vi "Get Robot Competition Mode.vi"(8 "Right Auton Limit":dbl, 9 "Right Teleop Limit":dbl, 10 "Finish":bool, 11 "DS Occurrence":refnum<k4>) -> (0 "Match Info out":T1={"Autonomous Elapsed Seconds"=0.0, "TeleOp Elapsed Seconds"=0.0, "Disabled Elapsed Seconds"=0.0, "Visited Autonomous"=FALSE, "Visited TeleOp"=FALSE, "Visited Disabled"=FALSE, "Autonomous Settings"={"Autonomous Style"=enum."Independent", "VI Refnum"=refnum}}, 1 "RawControlByte":u8 format="%08b", 2 "Call Context":T2, 3 "Robot Mode":T3, 4 "Right Limit":dbl)   [LabVIEW 2011]
doc: "<b>Get Competition Mode.vi</b> returns the mode of the current phase of competition, which determines the current restrictions of robot operation that apply. Possible modes include <b>Autonomous Disabled</b>, <b>Autonomous Enabled</b>, <b>Teleop Disabled</b>, and <b>Teleop Enabled</b>.\n\nThis software is licensed. Open the labview\\readme\\WPI Robotics Library Open Source License.txt file for more information."
uses:
  <vilib>/Rock Robotics/WPI/DriverStation/WPI_DriverStationRobotMode.ctl
  <vilib>/Rock Robotics/WPI/DriverStation/WPI_DriverStationDerivedRobotMode.ctl
  <vilib>/Rock Robotics/WPI/DriverStation/WPI_DriverStationMatch Info.ctl
  <vilib>/Rock Robotics/WPI/DriverStation/WPI_DriverStationCommDataCacheOp.ctl
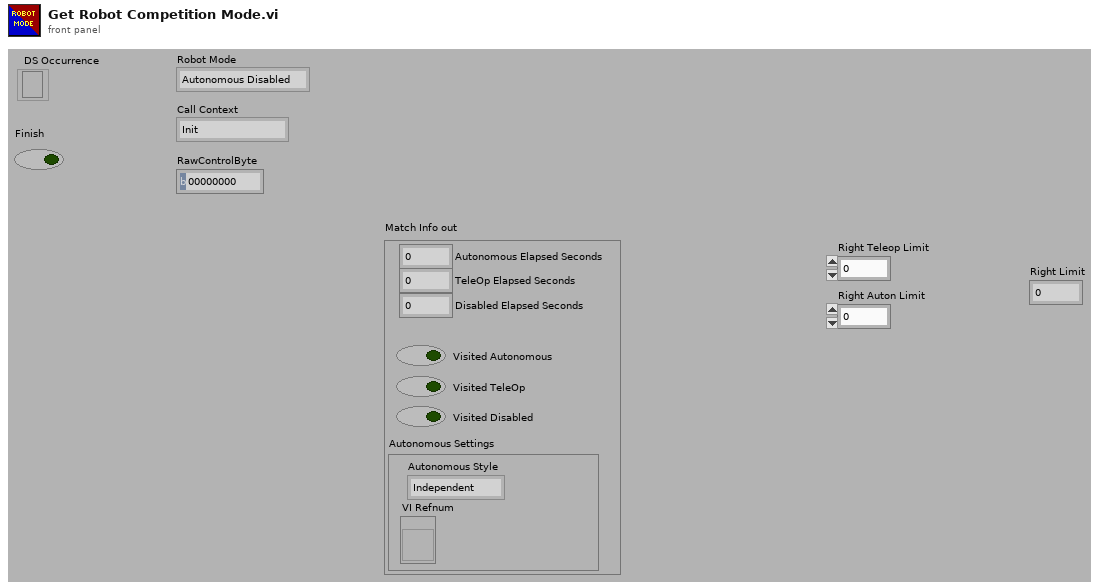
[diagram p1: front panel]
types:
  T1 = typedef "WPI_DriverStationMatch Info.ctl" = cluster{"Autonomous Elapsed Seconds":dbl, "TeleOp Elapsed Seconds":dbl, "Disabled Elapsed Seconds":dbl, "Visited Autonomous":bool, "Visited TeleOp":bool, "Visited Disabled":bool, "Autonomous Settings":cluster{"Autonomous Style":enum16{"Iterative", "Independent"}, "VI Refnum":refnum<vi>}}
  T2 = typedef "WPI_DriverStationDerivedRobotMode.ctl" = enum16{"Init", "Execute", "Stop"}
  T3 = typedef "WPI_DriverStationRobotMode.ctl" = enum16{"Autonomous Disabled", "Autonomous Enabled", "Teleop Disabled", "Teleop Enabled", "Timeout", "Finish"}
  T4 = typedef "WPI_DriverStationCommDataCacheOp.ctl" = enum16{"Get", "Set", "Init"}
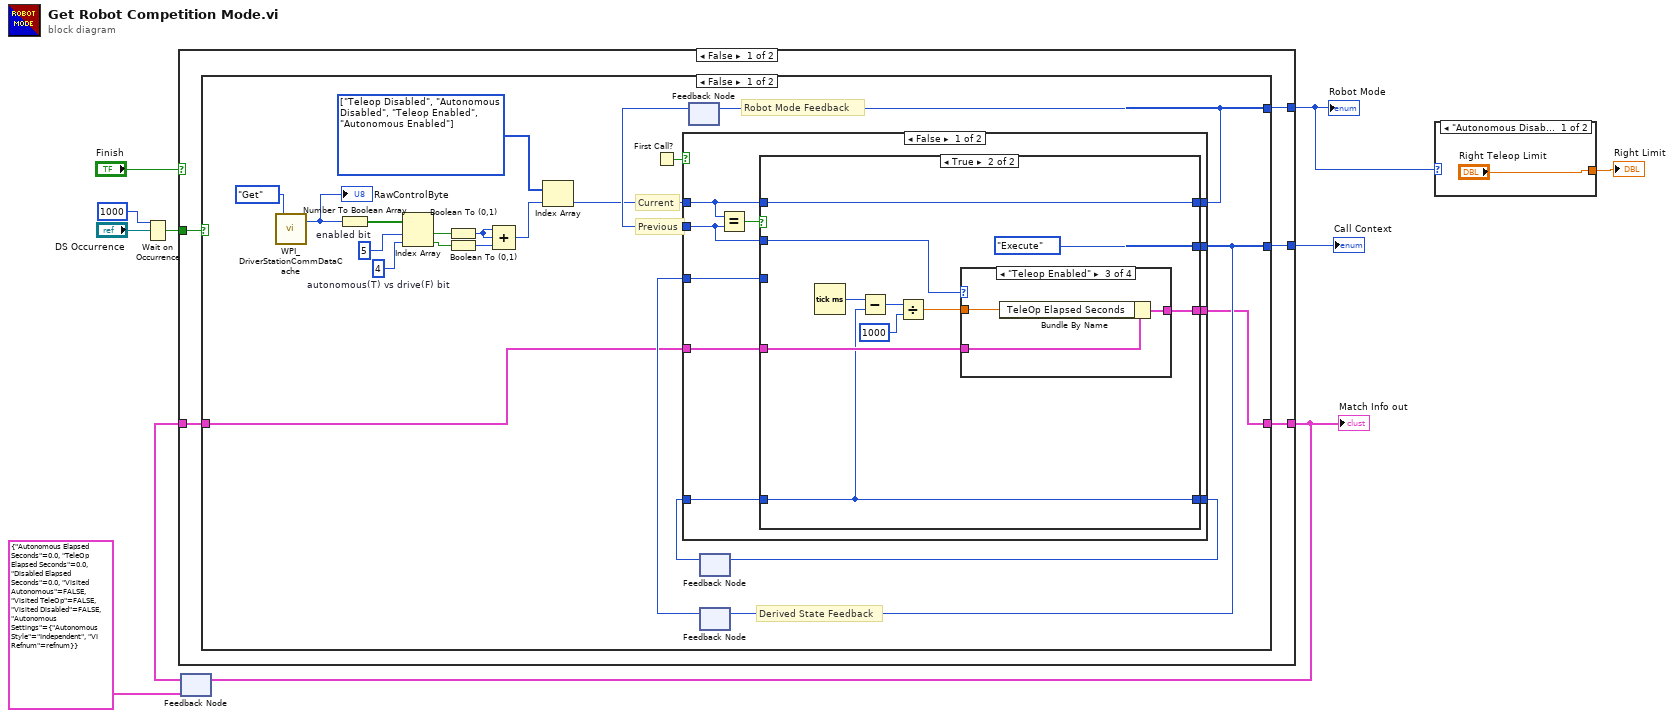
[diagram p0: block diagram]
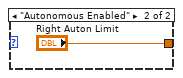
[diagram p2: hidden frame]
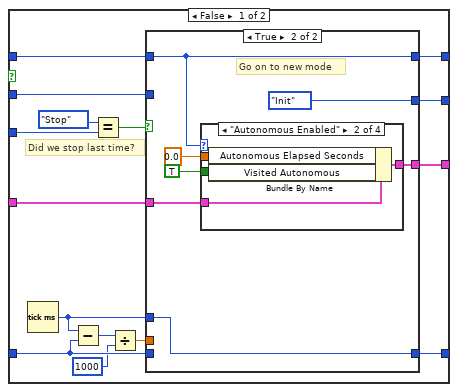
[diagram p3: hidden frame]
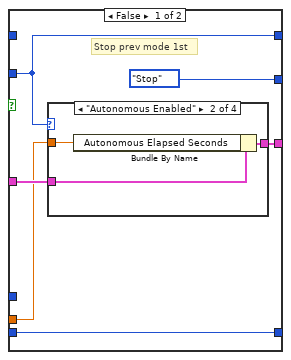
[diagram p4: hidden frame]
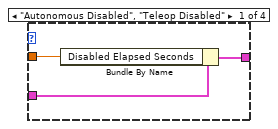
[diagram p5: hidden frame]
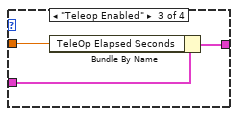
[diagram p6: hidden frame]
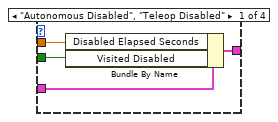
[diagram p8: hidden frame]
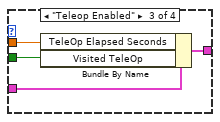
[diagram p9: hidden frame]
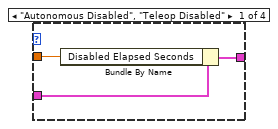
[diagram p11: hidden frame]
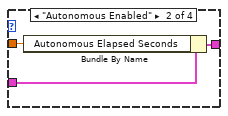
[diagram p12: hidden frame]
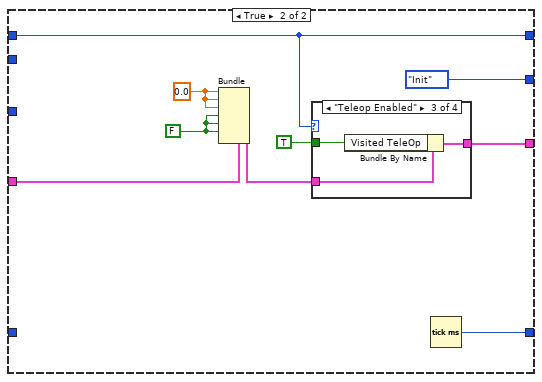
[diagram p14: hidden frame]
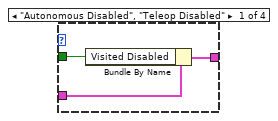
[diagram p15: hidden frame]
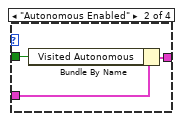
[diagram p16: hidden frame]
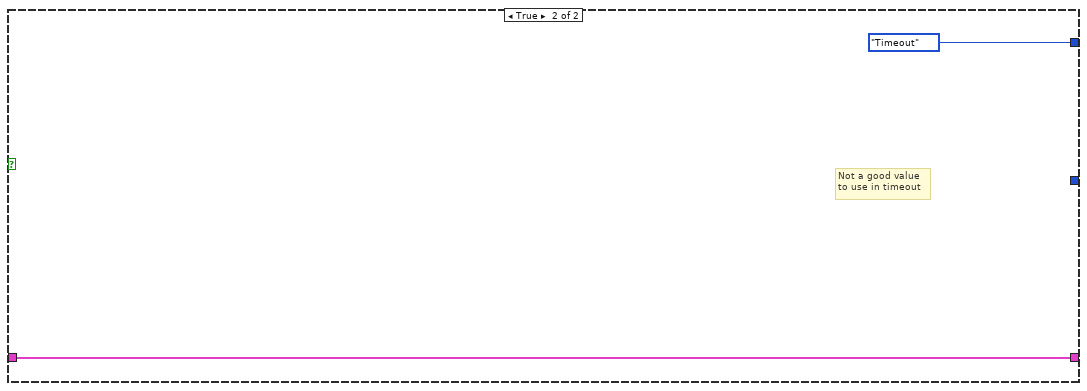
[diagram p18: hidden frame]
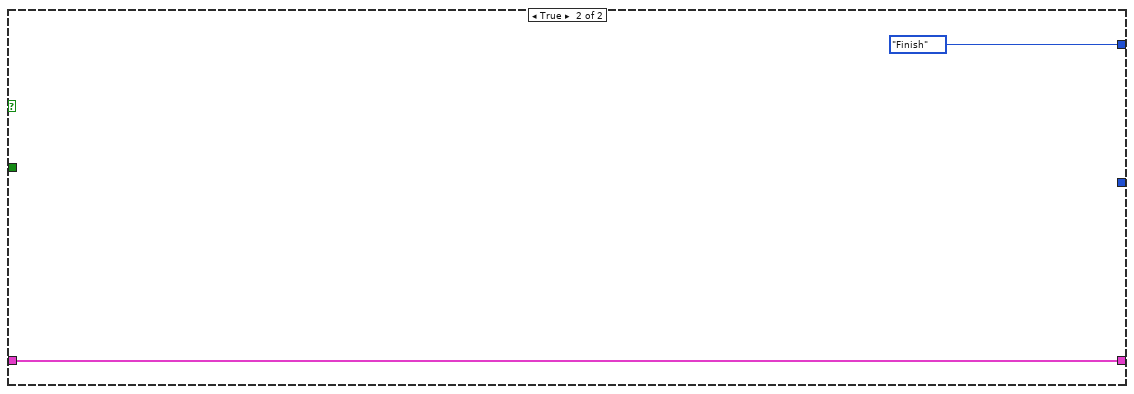
[diagram p19: hidden frame]
diagram:
  n1 = Wait on Occurrence(2:"DS Occurrence", 3:1000 ("ms timeout (-1)")) -> (0:w8:bool)  [unwired: 1 out]
  n2 = feedback #1(T1 {"Autonomous Elapsed Seconds"=0.0, "TeleOp Elapsed Seconds"=0.0, "Disabled Elapsed Seconds"=0.0, "Visited Autonomous"=FALSE, "Visited TeleOp"=FALSE, "Visited Disabled"=FALSE, "Autonomous Settings"={"Autonomous Style"=enum."Independent", "VI Refnum"=refnum}} ("Match Info")) -> (w4:T1)
  n3 = case shown="False" "Finish" {
    tunnel: [w15 _] -> w10
    tunnel: [w14 WPI_DriverStationRobotMode."Finish" ("RobotMode")] -> w2
    tunnel: w8 -> [w13 _]
    tunnel: w4 -> [w12 w139]
    tunnel: [w11 w139] -> w5
    frame False {
      n4 = case shown="False" w13 {
        tunnel: [w28 _] -> w15
        tunnel: [w27 WPI_DriverStationRobotMode."Timeout" ("RobotMode")] -> w14
        tunnel: w12 -> [w16 w137]
        tunnel: [w17 w137] -> w11
        frame False {
          w26 = T3[] [enum."Teleop Disabled", enum."Autonomous Disabled", enum."Teleop Enabled", enum."Autonomous Enabled"] items=["Autonomous Disabled", "Autonomous Enabled", "Teleop Disabled", "Teleop Enabled", "Timeout", "Finish"]
          w32 = 4  # autonomous(T) vs drive(F) bit
          w33 = 5  # enabled bit
          # "Derived State Feedback"
          # "Robot Mode Feedback"
          # "Previous"
          # "Current"
          n5 = call <vilib>:"WPI_DriverStationCommDataCache.vi"("CommDataCacheOp"=WPI_DriverStationCommDataCacheOp."Get") -> ("ControlBit out"=w35:u8)  [unwired: 18 out]
          "RawControlByte" <- w35
          n6 = Number To Boolean Array(number=w35) -> (Boolean array=w34:bool[])
          n7 = Index Array(array=w34, index #1=w33, index #2=w32) -> (element #1=w23:bool, element #2=w22:bool)
          n8 = Boolean To (0,1)(Boolean=w23) -> (0, 1=w25:i16)
          n9 = Boolean To (0,1)(Boolean=w22) -> (0, 1=w24:i16)
          n10 = Compound Arithmetic op=ADD(w25, w25, w24) -> (w21:i16)
          n11 = Index Array(array=w26, index=w21) -> (element=w20:T3)
          n12 = First Call?() -> (First Call?: T/F=w29:bool)
          n13 = feedback #2() -> (w30:T3)  [unwired: 1 out]
          n14 = feedback #3() -> (w18:u32)  [unwired: 1 out]
          n15 = feedback #4() -> (w31:T2)  [unwired: 1 out]
          n16 = case shown="False" w29 {
            tunnel: [w46 w118] -> w27
            tunnel: [w45 WPI_DriverStationDerivedRobotMode."Init" ("Derived Robot State")] -> w28
            tunnel: w31 -> [w43 _]
            tunnel: w20 -> [w42 w118]
            tunnel: w30 -> [w41 _]
            tunnel: w16 -> [w40 w125]
            tunnel: [w39 w120] -> w17
            tunnel: [w37 w122] -> w19
            tunnel: w18 -> [w38 _]
            frame False {
              n17 = Equal?(x=w42, y=w41) -> (x = y?=w44:bool)
              n18 = case shown="True" w44 {
                tunnel: w42 -> [w59 w107]
                tunnel: [w58 w107] -> w46
                tunnel: [w57 WPI_DriverStationDerivedRobotMode."Execute" ("Derived Robot State")] -> w45
                tunnel: w43 -> [w61 _]
                tunnel: w41 -> [w56 w102]
                tunnel: w40 -> [w50 w103]
                tunnel: [w54 w104] -> w39
                tunnel: w38 -> [w51 w101]
                tunnel: [w52 w101] -> w37
                frame False {
                  # "Did we stop last time?"
                  n19 = Tick Count (ms)() -> (millisecond timer value=w53:u32)
                  n20 = Subtract(x=w53, y=w51) -> (x-y=w49:u32)
                  n21 = Equal?(x=WPI_DriverStationDerivedRobotMode."Stop" ("Derived Robot State"), y=w61) -> (x = y?=w60:bool)
                  n22 = Divide(x=w49, y=1000) -> (x/y=w48:dbl)
                  n23 = case shown="True" w60 {
                    tunnel: w59 -> [_ w83]
                    tunnel: [w62 w83] -> w58
                    tunnel: [WPI_DriverStationDerivedRobotMode."Stop" ("Derived Robot State") WPI_DriverStationDerivedRobotMode."Init" ("Derived Robot State")] -> w57
                    tunnel: w56 -> [w62 _]
                    tunnel: w50 -> [w65 w81]
                    tunnel: [w66 w80] -> w54
                    tunnel: w48 -> [w64 _]
                    tunnel: w53 -> [_ w78]
                    tunnel: [w63 w78] -> w52
                    tunnel: w51 -> [w63 _]
                    frame False {
                      # "Stop prev mode 1st"
                      n24 = case shown="\"Autonomous Enabled\"" w62 {
                        tunnel: w64 -> [w70 w73 w76 _]
                        tunnel: w65 -> [w69 w72 w75 w77]
                        tunnel: [w68 w71 w74 w77] -> w66
                        frame "Autonomous Disabled", "Teleop Disabled" {
                          n25 = Bundle By Name(cluster=w69, "Disabled Elapsed Seconds"=w70) -> (w68:T1)
                        }
                        frame "Autonomous Enabled" {
                          n26 = Bundle By Name(cluster=w72, "Autonomous Elapsed Seconds"=w73) -> (w71:T1)
                        }
                        frame "Teleop Enabled" {
                          n27 = Bundle By Name(cluster=w75, "TeleOp Elapsed Seconds"=w76) -> (w74:T1)
                        }
                        frame Default {
                        }
                      }
                    }
                    frame True {
                      # "Go on to new mode"
                      n28 = case shown="\"Autonomous Enabled\"" w83 {
                        tunnel: 0.0 -> [w88 w92 w93 _]
                        tunnel: w81 -> [w87 w91 w96 w97]
                        tunnel: [w86 w90 w95 w97] -> w80
                        tunnel: TRUE -> [w85 w89 w94 _]
                        frame "Autonomous Disabled", "Teleop Disabled" {
                          n29 = Bundle By Name(cluster=w87, "Disabled Elapsed Seconds"=w88, "Visited Disabled"=w85) -> (w86:T1)
                        }
                        frame "Autonomous Enabled" {
                          n30 = Bundle By Name(cluster=w91, "Autonomous Elapsed Seconds"=w92, "Visited Autonomous"=w89) -> (w90:T1)
                        }
                        frame "Teleop Enabled" {
                          n31 = Bundle By Name(cluster=w96, "TeleOp Elapsed Seconds"=w93, "Visited TeleOp"=w94) -> (w95:T1)
                        }
                        frame Default {
                        }
                      }
                    }
                  }
                }
                frame True {
                  n32 = Tick Count (ms)() -> (millisecond timer value=w105:u32)
                  n33 = Subtract(x=w105, y=w101) -> (x-y=w99:u32)
                  n34 = Divide(x=w99, y=u32 1000) -> (x/y=w100:dbl)
                  n35 = case shown="\"Teleop Enabled\"" w102 {
                    tunnel: w100 -> [w110 w113 w116 _]
                    tunnel: w103 -> [w109 w112 w115 w117]
                    tunnel: [w108 w111 w114 w117] -> w104
                    frame "Autonomous Disabled", "Teleop Disabled" {
                      n36 = Bundle By Name(cluster=w109, "Disabled Elapsed Seconds"=w110) -> (w108:T1)
                    }
                    frame "Autonomous Enabled" {
                      n37 = Bundle By Name(cluster=w112, "Autonomous Elapsed Seconds"=w113) -> (w111:T1)
                    }
                    frame "Teleop Enabled" {
                      n38 = Bundle By Name(cluster=w115, "TeleOp Elapsed Seconds"=w116) -> (w114:T1)
                    }
                    frame Default {
                    }
                  }
                }
              }
            }
            frame True {
              w124 = 0.0
              w123 = FALSE
              n39 = Bundle(cluster=w125, "Autonomous Elapsed Seconds"=w124, "TeleOp Elapsed Seconds"=w124, "Disabled Elapsed Seconds"=w124, "Visited Autonomous"=w123, "Visited TeleOp"=w123, "Visited Disabled"=w123) -> (w121:T1)  [unwired: 1 out]
              n40 = case shown="\"Teleop Enabled\"" w118 {
                tunnel: w121 -> [w129 w132 w135 w136]
                tunnel: [w128 w131 w134 w136] -> w120
                tunnel: TRUE -> [w127 w130 w133 _]
                frame "Autonomous Disabled", "Teleop Disabled" {
                  n41 = Bundle By Name(cluster=w129, "Visited Disabled"=w127) -> (w128:T1)
                }
                frame "Autonomous Enabled" {
                  n42 = Bundle By Name(cluster=w132, "Visited Autonomous"=w130) -> (w131:T1)
                }
                frame "Teleop Enabled" {
                  n43 = Bundle By Name(cluster=w135, "Visited TeleOp"=w133) -> (w134:T1)
                }
                frame Default {
                }
              }
              n44 = Tick Count (ms)() -> (millisecond timer value=w122:u32)
            }
          }
          n45 = feedback-in #2(w27) -> ()
          n46 = feedback-in #3(w19) -> ()
          n47 = feedback-in #4(w28) -> ()
        }
        frame True {
          # "Not a good value\nto use in timeout"
        }
      }
    }
    frame True {
    }
  }
  "Robot Mode" <- w2
  "Call Context" <- w10
  "Match Info out" <- w5
  n48 = feedback-in #1(w5) -> ()
  n49 = case shown="\"Autonomous Disabled\", Default" w2 {
    tunnel: ["Right Teleop Limit" "Right Auton Limit"] -> w1
    frame "Autonomous Disabled", Default {
    }
    frame "Autonomous Enabled" {
    }
  }
  "Right Limit" <- w1
